vi "Functional Global.vi"(7 "Commande":T1, 8 "entrée d'erreur (pas d'erreur)":errorcluster) -> (0 "sortie d'erreur":errorcluster, 2 "Compte":i32 caption="Nombre")   [LabVIEW 2009]
uses:
  Functional Global Command.ctl
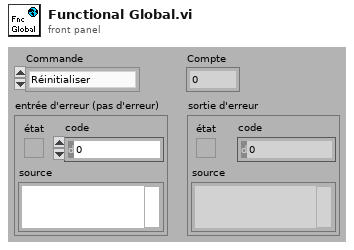
[diagram p1: front panel]
types:
  T1 = typedef "Functional Global Command.ctl" = enum16{"Réinitialiser", "Incrémenter", "Obtenir le compte"}
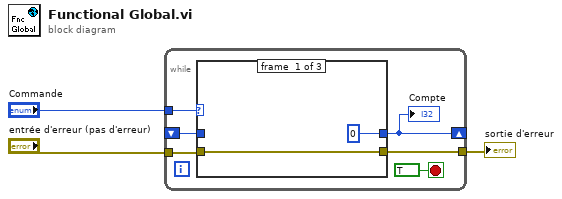
[diagram p0: block diagram]
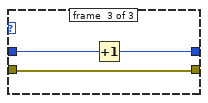
[diagram p3: hidden frame]
diagram:
  n1 = while "Boucle While" {
    tunnel: "Commande" -> [w8]
    shift-right: [w6] -> _
    shift-left: _ -> [w7]
    tunnel: "entrée d'erreur (pas d'erreur)" -> [w5]
    tunnel: [w4] -> w1
    stop <- TRUE stop-if-true
    n2 = case "Structure Condition" shown="\"Obtenir le compte\", Par défaut" w8 {
      tunnel: [0 w13 w15] -> w6
      tunnel: w7 -> [_ w13 w16]
      tunnel: [w10 w12 w14] -> w4
      tunnel: w5 -> [w10 w12 w14]
      frame #0 {
      }
      frame #1 {
      }
      frame #2 {
        n3 = Increment(x=w16) -> (x+1=w15:i32)
      }
    }
    "Compte" <- w6
  }
  "sortie d'erreur" <- w1
